vi "Pose3d_Interpolate.vi"(9 "T":dbl, 10 "EndValue Pose3d":T1={"Translation3d"={"X"=0.0, "Y"=0.0, "Z"=0.0}, "Rotation3d"={"Q_quaternion"={"R"=1.0, "V"=[0.0, 0.0, 0.0]}}} {"Translation3d"."Z" format="%14.3f"; "Translation3d"."Y" format="%14.3f"; "Translation3d"."X" format="%14.3f"}, 11 "in Pose3d":T1={"Translation3d"={"X"=0.0, "Y"=0.0, "Z"=0.0}, "Rotation3d"={"Q_quaternion"={"R"=1.0, "V"=[0.0, 0.0, 0.0]}}} {"Translation3d"."Z" format="%14.3f"; "Translation3d"."Y" format="%14.3f"; "Translation3d"."X" format="%14.3f"}) -> (3 "Interpolated Pose3d":T1={"Translation3d"={"X"=0.0, "Y"=0.0, "Z"=0.0}, "Rotation3d"={"Q_quaternion"={"R"=1.0, "V"=[0.0, 0.0, 0.0]}}} {"Translation3d"."Z" format="%14.3f"; "Translation3d"."Y" format="%14.3f"; "Translation3d"."X" format="%14.3f"})   [LabVIEW 2019, in "Trajectory_Library.lvlib"]
doc: "Interpolate between 2 poses\n\nParameter:\n - IN POSE3D - Current POSE data structure\n - EndValue POSE3D -- The end value POSE..\n - T -- Value between 0 and 1. \n\nReturns:\n - Interpolated POSE3D - The interpolated POSE."
uses:
  Trajectory_Library.lvlib
  TypeDef/TRANSLATION3D.ctl
  TypeDef/QUATERNION.ctl
  TypeDef/ROTATION3D.ctl
  TypeDef/POSE3D.ctl
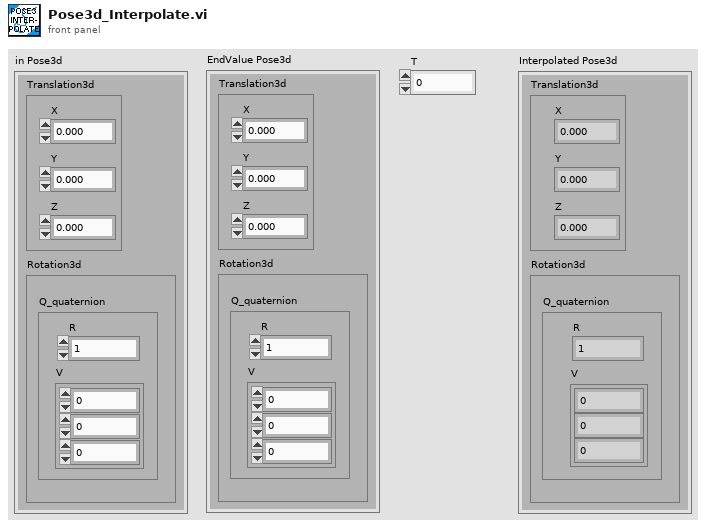
[diagram p1: front panel]
types:
  T1 = typedef "Trajectory_Library.lvlib/POSE3D.ctl" = cluster{"Translation3d":T2, "Rotation3d":T3}
  T2 = typedef "Trajectory_Library.lvlib/TRANSLATION3D.ctl" = cluster{"X":dbl, "Y":dbl, "Z":dbl}
  T3 = typedef "Trajectory_Library.lvlib/ROTATION3D.ctl" = cluster{"Q_quaternion":T4}
  T4 = typedef "Trajectory_Library.lvlib/QUATERNION.ctl" = cluster{"R":dbl, "V":dbl[]}
  T5 = typedef "WPILib_Math.lvlib/TWIST3D.ctl" = cluster{"dX":dbl, "dY":dbl, "dZ":dbl, "rX":dbl, "rY":dbl, "rZ":dbl}
  T6 = typedef "Trajectory_Library.lvlib/TWIST3D.ctl" = cluster{"dX":dbl, "dY":dbl, "dZ":dbl, "rX":dbl, "rY":dbl, "rZ":dbl}
  T7 = typedef "WPILib_Math.lvlib/POSE3D.ctl" = cluster{"Translation3d":T8, "Rotation3d":T9}
  T8 = typedef "WPILib_Math.lvlib/TRANSLATION3D.ctl" = cluster{"X":dbl, "Y":dbl, "Z":dbl}
  T9 = typedef "WPILib_Math.lvlib/ROTATION3D.ctl" = cluster{"Q_quaternion":T10}
  T10 = typedef "WPILib_Math.lvlib/QUATERNION.ctl" = cluster{"R":dbl, "V":dbl[]}
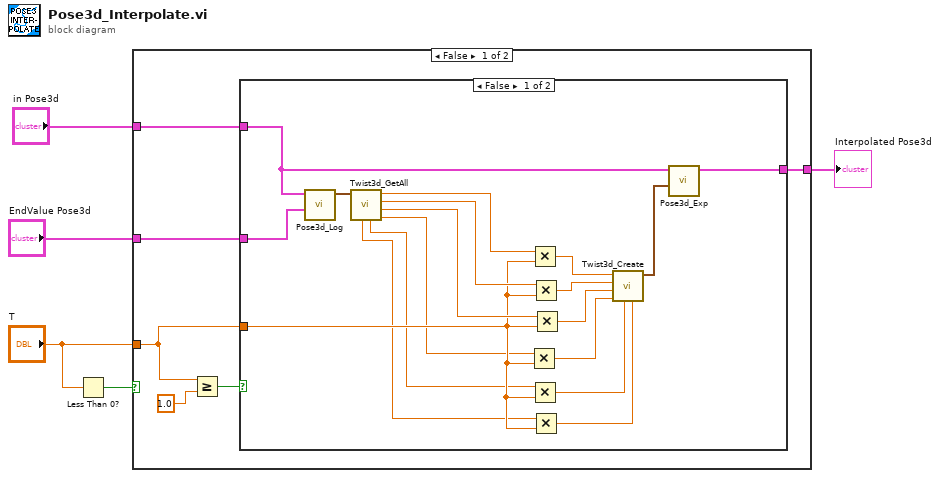
[diagram p0: block diagram]
diagram:
  n1 = Less Than 0?(x="T") -> (x < 0?=w5:bool)
  n2 = case shown="False" w5 {
    tunnel: "T" -> [w6 _]
    tunnel: [w8 w31] -> w3
    tunnel: "in Pose3d" -> [w7 w31]
    tunnel: "EndValue Pose3d" -> [w9 _]
    frame False {
      n3 = Greater Or Equal?(x=w6, y=1.0) -> (x >= y?=w10:bool)
      n4 = case shown="False" w10 {
        tunnel: w9 -> [w29 w30]
        tunnel: [w19 w30] -> w8
        tunnel: w7 -> [w21 _]
        tunnel: w6 -> [w18 _]
        frame False {
          n5 = call "Pose3d_Log.vi"("end Pose3d"=w29, "in Pose3d"=w21) -> ("out Twist3d"=w28:T5)  [unwired: 9 in]
          n6 = call "Twist3d_GetAll.vi"("Twist3d"=w28) -> ("rX"=w17:dbl, "dZ"=w25:dbl, "dY"=w26:dbl, "dX"=w27:dbl, "rY"=w16:dbl, "rZ"=w15:dbl)  [unwired: 5 in]
          n7 = Multiply(x=w17, y=w18) -> (x*y=w14:dbl)
          n8 = Multiply(x=w27, y=w18) -> (x*y=w24:dbl)
          n9 = Multiply(x=w16, y=w18) -> (x*y=w13:dbl)
          n10 = Multiply(x=w26, y=w18) -> (x*y=w23:dbl)
          n11 = Multiply(x=w15, y=w18) -> (x*y=w12:dbl)
          n12 = Multiply(x=w25, y=w18) -> (x*y=w22:dbl)
          n13 = call "Twist3d_Create.vi"("rZ"=w12, "rY"=w13, "rX"=w14, "dZ"=w22, "dY"=w23, "dX"=w24) -> ("Twist3d"=w20:T6)  [unwired: 5 in]
          n14 = call "Pose3d_Exp.vi"("Twist3d"=w20, "Pose3d"=w21) -> ("Updated Pose3d"=w19:T7)  [unwired: 9 in]
        }
        frame True {
        }
      }
    }
    frame True {
    }
  }
  "Interpolated Pose3d" <- w3
